vi "Write Sound File Path.vi"(8 "error in (no error)":errorcluster, 10 "Sound File Path":path=path "../support/sample.wav", 11 "Sounds in":refnum<class "Sounds.lvclass">) -> (0 "error out":errorcluster, 3 "Sounds out":refnum<class "Sounds.lvclass">)   [LabVIEW 2021, in "Sounds.lvlib" / "Sounds.lvclass"]
uses:
  Sounds.lvclass
  Sounds.lvclass/Sounds.ctl
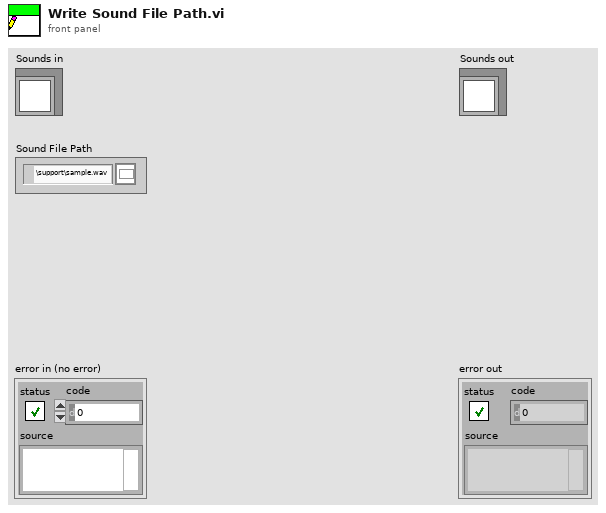
[diagram p1: front panel]
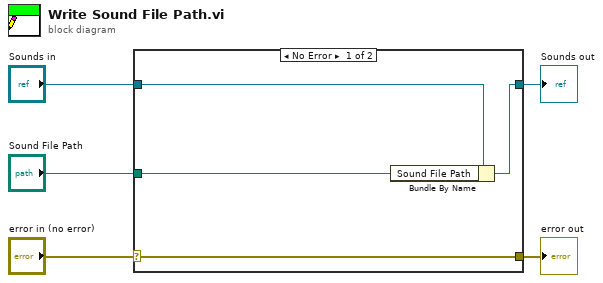
[diagram p0: block diagram]
diagram:
  n1 = case shown="No Error" "error in (no error)" {
    selector: "error in (no error)" -> [w9 w10]
    tunnel: [w9 w10] -> w4
    tunnel: [w7 w11] -> w2
    tunnel: "Sounds in" -> [w8 w11]
    tunnel: "Sound File Path" -> [w6 _]
    frame No Error {
      n2 = Bundle By Name(cluster=w8, "Sound File Path"=w6) -> (w7:refnum<class "Sounds.lvclass">)
    }
    frame Error {
    }
  }
  "error out" <- w4
  "Sounds out" <- w2
